vi "Format Entry.vi"(8 "error in (no error)":errorcluster, 10 "Log Data":T1={"Time"=timestamp(0 s since 1904-01-01), "Level"=enum."INFO", "Logger"="", "Message"="", "Arguments"=[]} {"Time" format="%<%x %.3X>T"}, 11 "DBLayout in":refnum<class "DBLayout.lvclass">) -> (0 "error out":errorcluster, 2 "Log Entry":string, 3 "DBLayout out":refnum<class "DBLayout.lvclass">)   [LabVIEW 2019, in "TSC Event Logger.lvlib" / "DBLayout.lvclass"]
uses:
  DBLayout.lvclass
  Log Data.ctl
  Log/Event Level.ctl
  Layout.lvclass
  TSC Event Logger.lvlib
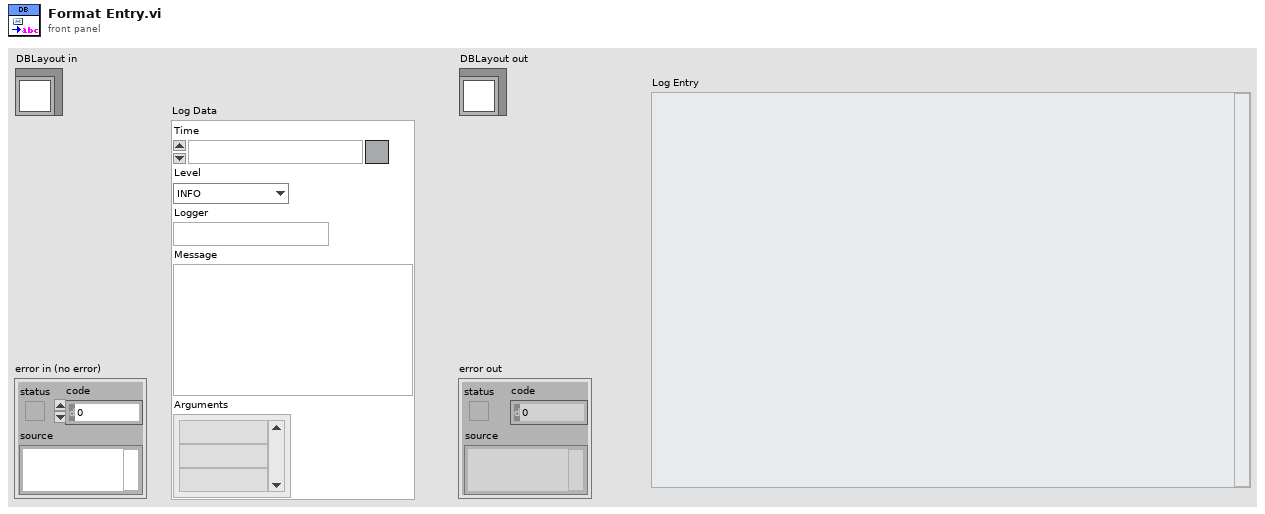
[diagram p1: front panel]
types:
  T1 = typedef "TSC Event Logger.lvlib/Log Data.ctl" = cluster{"Time":timestamp, "Level":T2, "Logger":string, "Message":string, "Arguments":string[]}
  T2 = typedef "TSC Event Logger.lvlib/Event Level.ctl" = enum16{"OFF", "TRACE", "DEBUG", "INFO", "WARN", "ERROR", "FATAL"}
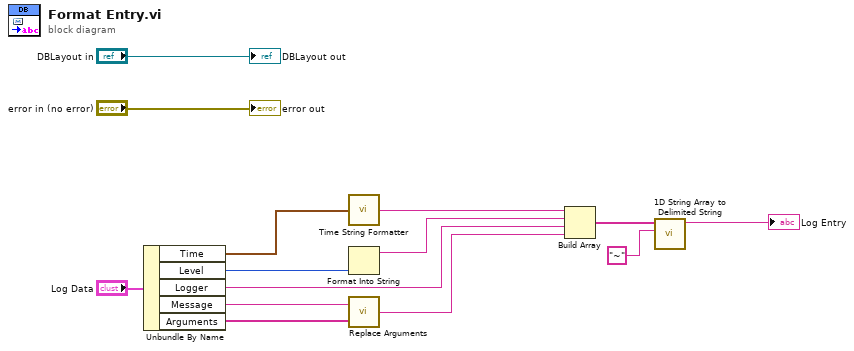
[diagram p0: block diagram]
diagram:
  n1 = Unbundle By Name("Log Data") -> ("Time"=w12:timestamp, "Level"=w11:T2, "Logger"=w7:string, "Message"=w6:string, "Arguments"=w5:string[])
  n2 = call "Time String Formatter.vi"("Time"=w12) -> ("Time string"=w9:string)
  n3 = Format Into String(w11) -> (resulting string=w8:string)  [unwired: 3 in, 1 out]
  n4 = call "Replace Arguments.vi"("Arguments"=w5, "Message"=w6) -> ("Output Message"=w4:string)
  n5 = Build Array(w9, w8, w7, w4) -> (w3:string[])
  n6 = call <vilib>:"1D String Array to Delimited String.vi"("delimiter"="~", "string array"=w3) -> ("delimited string"=→"Log Entry":string)  [unwired: 9 in]
  "error out" <- "error in (no error)"
  "DBLayout out" <- "DBLayout in"
